vi "直通基准_开始消息.vi"(9 "COM":i32, 10 "A":i32) -> ()   [LabVIEW 2015]
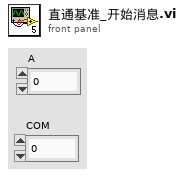
[diagram p1: front panel]
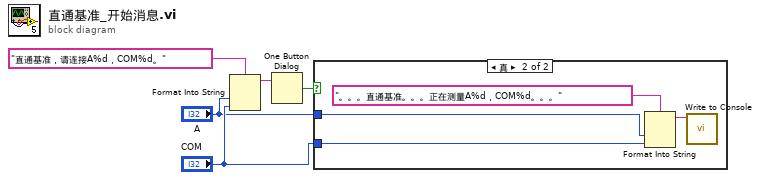
[diagram p0: block diagram]
diagram:
  n1 = Format Into String(format string="直通基准，请连接A%d，COM%d。", "A", "COM") -> (resulting string=w4:string)  [unwired: 2 in, 1 out]
  n2 = One Button Dialog(message=w4) -> (true=w5:bool)  [unwired: 1 in]
  n3 = case shown="真" w5 {
    tunnel: "A" -> [_ w8]
    tunnel: "COM" -> [_ w7]
    frame False {
    }
    frame True {
      n4 = Format Into String(format string="。。。直通基准。。。正在测量A%d，COM%d。。。", w8, w7) -> (resulting string=w6:string)  [unwired: 2 in, 1 out]
      n5 = call "Write to Console.vi"("Input"=w6) -> ()  [unwired: 10 in, 1 out]
    }
  }
